vi "HP 5890 Serial Port Init.vi"(5 "flow control etc.":T1={"input XON/XOFF"=TRUE, "input HW Handshake"=FALSE, "input alt HW HShk"=FALSE, "output XON/XOFF"=TRUE, "output HW Handshake"=FALSE, "output alt HW HShk"=FALSE, "XOFF byte "=19, "XON byte"=17, "parity error byte"=0} {"parity error byte" format="%.0x"; "XON byte" format="%.0x"; "XOFF byte" format="%.0x"}, 6 "parity":u16(ring) items=["no parity", "odd parity", "even parity", "mark parity", "space parity"], 8 "stop bits":u16(ring) items=["1 bit", "1.5 bits", "2 bits"], 9 "data bits":u16=8 min=5 max=8 step=1, 10 "baud rate":u16=19200, 11 "port number":refnum<visa-resource-name>) -> (0 "timed out":bool, 4 "error code":i32)   [LabVIEW 2012]
doc: "Initializes the selected serial port to the specified settings."
uses:
  <vilib>/Instr/_visa.llb/VISA Configure Serial Port (Instr).vi
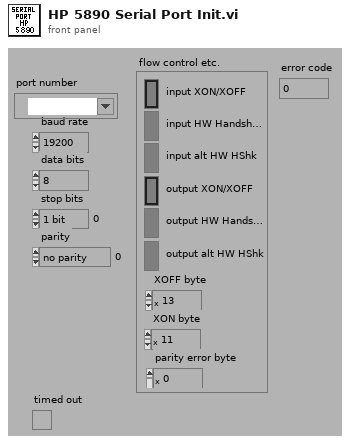
[diagram p1: front panel]
types:
  T1 = cluster{"input XON/XOFF":bool, "input HW Handshake":bool, "input alt HW HShk":bool, "output XON/XOFF":bool, "output HW Handshake":bool, "output alt HW HShk":bool, "XOFF byte ":u8, "XON byte":u8, "parity error byte":u16}
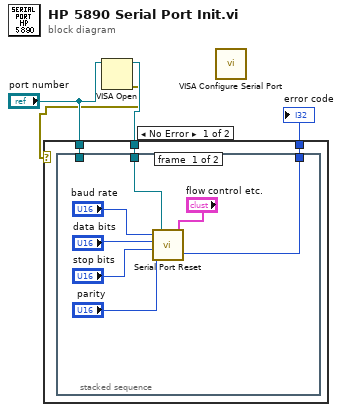
[diagram p0: block diagram]
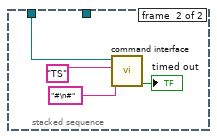
[diagram p2: hidden frame]
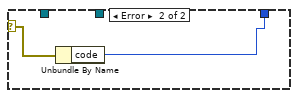
[diagram p3: hidden frame]
diagram:
  n1 = VISA Open(VISA resource name="port number") -> (VISA resource name=w2:refnum<visa-resource-name>, error out=w1:errorcluster)  [unwired: 4 in]
  n2 = case shown="No Error" w1 {
    selector: w1 -> [_ w20]
    tunnel: w2 -> [w7 _]
    tunnel: [w6 w19] -> w4
    tunnel: "port number" -> [w5 _]
    frame No Error {
      n3 = stacked-sequence {
        tunnel: w7 -> [w14 _]
        tunnel: [w10 _] -> w6
        tunnel: w5 -> [_ w18]
        frame #0 {
          n4 = call <vilib>:"Serial Port Reset.vi"("flow control etc."="flow control etc.", "input refnum"=w14, "parity"="parity", "stop bits"="stop bits", "data bits"="data bits", "baud rate"="baud rate") -> ("error"=w10:i32)  [unwired: 1 in]
        }
        frame #1 {
          n5 = call "command interface.vi"("Parameter"="#\n#", "command"="TS", "Serial Port"=w18) -> ("timed out"=→"timed out":bool)  [unwired: 4 in, 3 out]
        }
      }
    }
    frame Error {
      n6 = Unbundle By Name(w20) -> ("code"=w19:i32)
    }
  }
  "error code" <- w4
  n7 = call-poly "VISA Configure Serial Port"() -> ()  [unwired: 14 in, 2 out]
